vi "DeviceOff.vi"(8 "error in (no error)":errorcluster, 11 "NhRegenGridSim in":refnum<class "NhRegenGridSim.lvclass">) -> (0 "error out":errorcluster, 3 "NhRegenGridSim out":refnum<class "NhRegenGridSim.lvclass">)   [LabVIEW 2018, in "AcPwrPlugins.lvlib" / "NhRegenGridSim.lvclass"]
doc: "This VI (if the unit is not already off) turns off the unit. Off is defined as the output relay being open."
uses:
  NhRegenGridSim.lvclass
  C:/Users/ico/Documents/Projects/NistPluggableModules/AcPwr/AcPwrPlugins/AcPwrBaseClass/AcPwrBase.lvclass
  AcPwrBaseClass/AcPwrBase.lvclass/AcPwrBase.ctl
  AcPwrBaseClass/Accessors/Read Phases.vi
  <instrlib>/NH Research 9400 Series/NH Research 9400 Series.lvlib
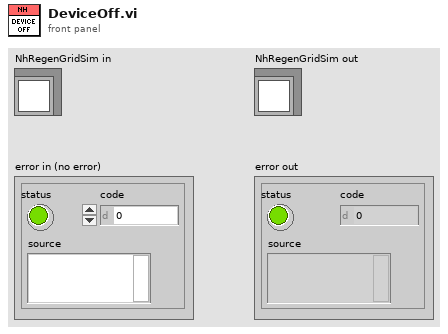
[diagram p1: front panel]
types:
  T1 = typedef "AcPwrPlugins.lvlib/AcPwrBase.lvclass/Phase.ctl" = cluster{"Name":string, "Enabled":bool, "VoltageLevel":dbl, "Handle":string, "VoltageRange":dbl[], "Connected":bool, "CurrentLimit":dbl, "Waveform":string}
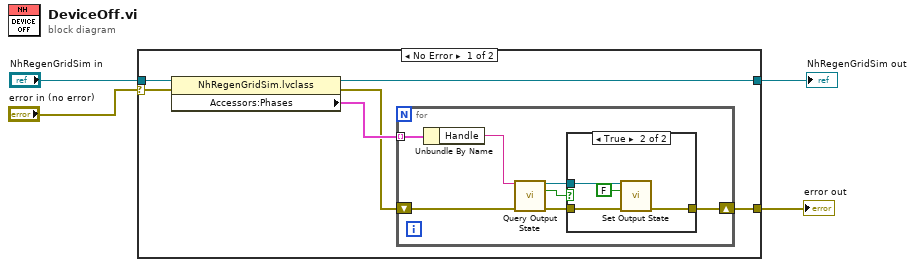
[diagram p0: block diagram]
diagram:
  n1 = case shown="No Error" "error in (no error)" {
    selector: "error in (no error)" -> [w6 w24]
    tunnel: [w8 w24] -> w4
    tunnel: [w7 w23] -> w3
    tunnel: "NhRegenGridSim in" -> [w5 w23]
    frame No Error {
      n2 = property class="NhRegenGridSim.lvclass"(reference=w5, error in=w6) -> (reference out=w7:refnum<class "NhRegenGridSim.lvclass">, error out=w9:errorcluster, "Accessors:Phases"=w10:T1[])
      n3 = for {
        tunnel: w10 -> [w17] mode=indexing
        shift-right: [w13] -> w8
        shift-left: w9 -> [w16]
        n4 = Unbundle By Name(w17) -> ("Handle"=w12:string)
        n5 = call <instrlib>:"Query Output State.vi"("VISA resource name"=w12, "error in (no error)"=w16) -> ("VISA resource name out"=w11:refnum<visa-resource-name>, "Output Enabled"=w15:bool, "error out"=w14:errorcluster)  [unwired: 11 in]
        n6 = case shown="True" w15 {
          tunnel: w14 -> [w18 w22]
          tunnel: [w18 w21] -> w13
          tunnel: w11 -> [_ w20]
          frame False {
          }
          frame True {
            n7 = call <instrlib>:"Set Output State.vi"("VISA resource name"=w20, "Output State (F: Disable)"=FALSE, "error in (no error)"=w22) -> ("error out"=w21:errorcluster)  [unwired: 11 in, 1 out]
          }
        }
      }
    }
    frame Error {
    }
  }
  "error out" <- w4
  "NhRegenGridSim out" <- w3
